vi "Set.vi"(6 "Labels":map{string, string}(c390), 8 "error in (no error)":errorcluster, 10 "Value":dbl, 11 "Gauge Ref":refnum<data-value>) -> (0 "error out":errorcluster, 3 "Gauge Ref out":refnum<data-value>)   [LabVIEW 2020, in "Metrics.lvlib" / "Gauge.lvclass"]
uses:
  Gauge.lvclass
  C:/Github-locals/PromVIEW/src/metrics/metric/Metric.lvclass
  metric/Metric.lvclass/Metric.ctl
  metric/Read Samples.vi
  metric/Read Name.vi
  metric/Write Samples.vi
  sample/Sample.lvclass
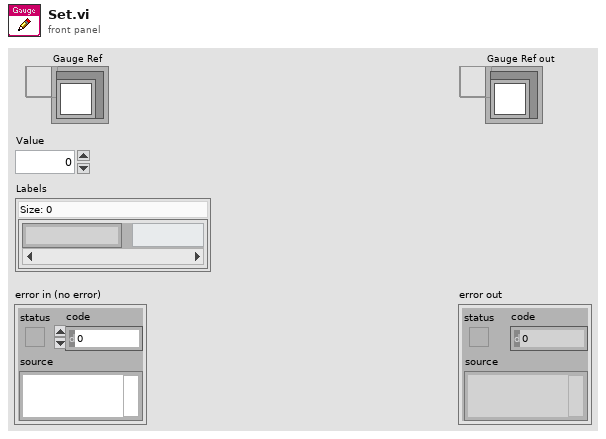
[diagram p1: front panel]
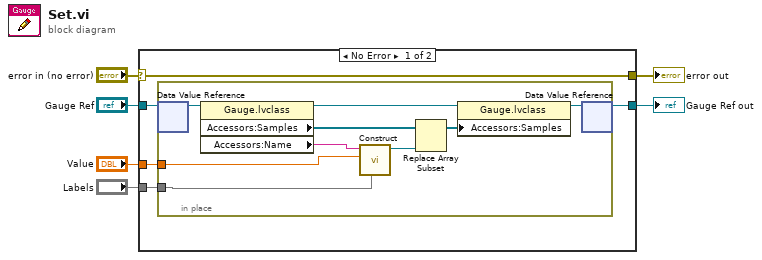
[diagram p0: block diagram]
diagram:
  n1 = case shown="No Error" "error in (no error)" {
    selector: "error in (no error)" -> [w11 w21]
    tunnel: [w11 w21] -> w5
    tunnel: "Gauge Ref" -> [w10 _]
    tunnel: "Value" -> [w9 _]
    tunnel: "Labels" -> [w8 _]
    tunnel: [w7 _] -> w1
    frame No Error {
      n2 = in-place {
        in-place-border: w9 -> [w13]
        in-place-border: w8 -> [w12]
        n3 = in-place-dvr #1(w10) -> (w20:refnum<class "Gauge.lvclass">)  [unwired: 1 out]
        n4 = property class="Gauge.lvclass"(reference=w20) -> (reference out=w17:refnum<class "Gauge.lvclass">, "Accessors:Samples"=w19:refnum<class "Sample.lvclass">[], "Accessors:Name"=w15:string)  [unwired: 1 in, 1 out]
        n5 = call "Construct.vi"("Labels"=w12, "Value"=w13, "Name"=w15) -> ("Sample out"=w14:refnum<class "Sample.lvclass">)  [unwired: 7 in, 1 out]
        n6 = Replace Array Subset(array=w19, new element=w14) -> (w18:refnum<class "Sample.lvclass">[])  [unwired: 1 in]
        n7 = property class="Gauge.lvclass"(reference=w17, "Accessors:Samples"=w18) -> (reference out=w16:refnum<class "Gauge.lvclass">)  [unwired: 1 in, 1 out]
        n8 = in-place-dvr #1(w16) -> (w7:refnum<data-value>)  [unwired: 1 out]
      }
    }
    frame Error {
    }
  }
  "error out" <- w5
  "Gauge Ref out" <- w1
